vi "Facade.vi"(0 "Data In":T4, 2 "Display State In":T2, 3 "Container State":T3) -> (6 "Data Out":T4, 7 "Display State Out":T2, 8 "Action":T1)   [LabVIEW 2009, in "HistoryPath.xctl"]
uses:
  HistoryPath.xctl
  Data.ctl
  <vilib>/_xctls/Container State.ctl
  State.ctl
  <vilib>/_xctls/Action.ctl
  <vilib>/_xctls/XControlSupport.lvlib
panel:
  in  "Browse":bool
  in  "Combo Box":string(combo)
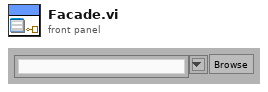
[diagram p1: front panel]
types:
  T1 = typedef "XControlSupport.lvlib/Action.ctl" = cluster{"Data Changed?":bool, "State Changed?":bool, "Action Name":string}
  T2 = typedef "HistoryPath.xctl/State.ctl" = cluster{"History":path[], "History Length":i32}
  T3 = typedef "XControlSupport.lvlib/Container State.ctl" = cluster{"Indicator?":bool, "Run Mode?":bool, " Refnum":refnum<vi>}
  T4 = typedef "HistoryPath.xctl/Data.ctl" = path
  T5 = enum8{"Enabled", "Disabled", "Disabled and Grayed Out"}
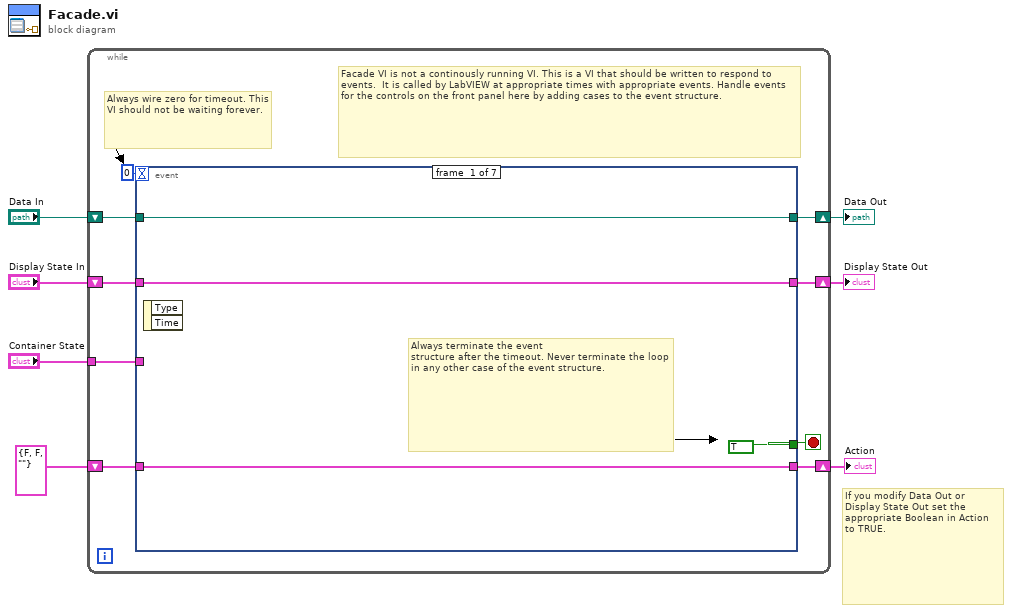
[diagram p0: block diagram]
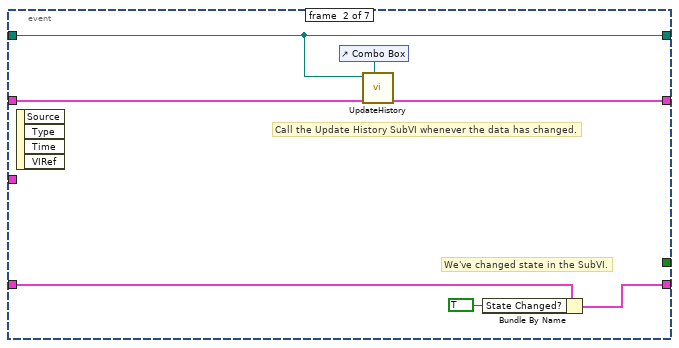
[diagram p2: hidden frame]
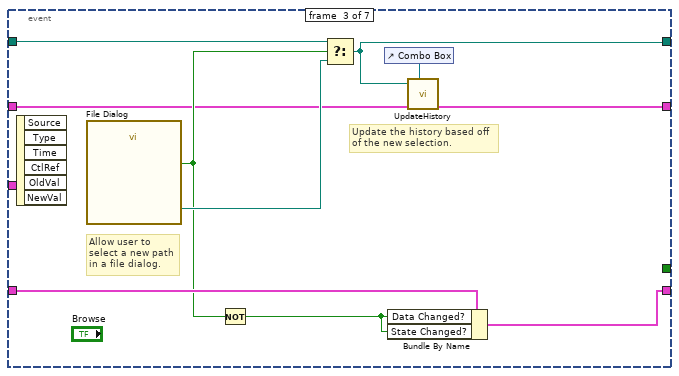
[diagram p3: hidden frame]
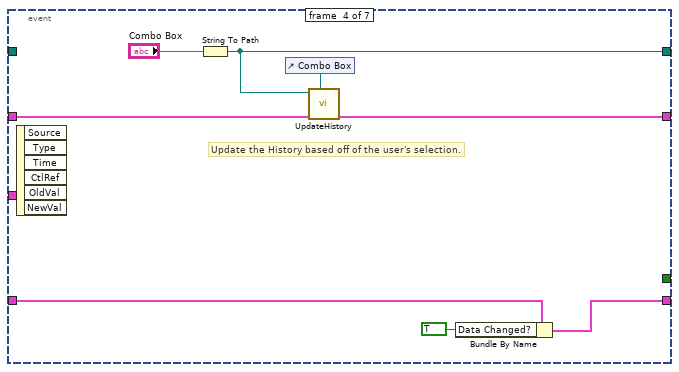
[diagram p4: hidden frame]
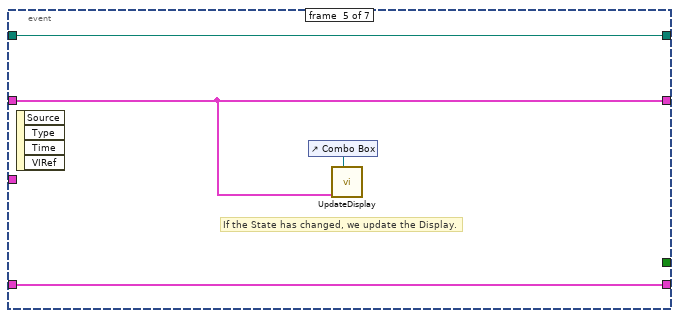
[diagram p5: hidden frame]
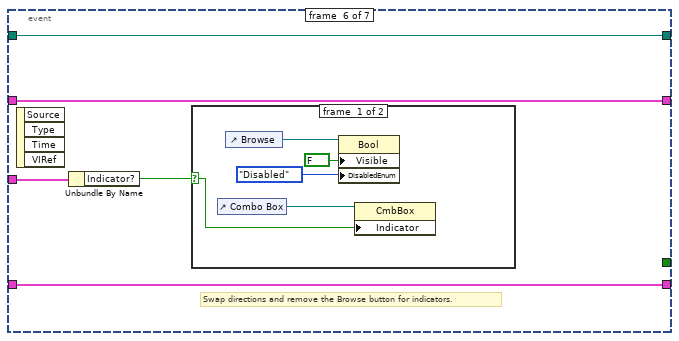
[diagram p6: hidden frame]
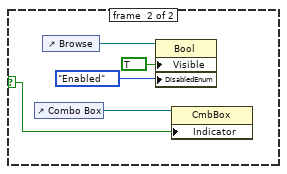
[diagram p7: hidden frame]
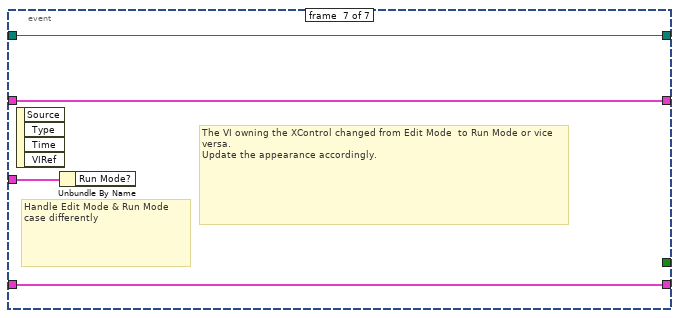
[diagram p8: hidden frame]
diagram:
  # "If you modify Data Out or\nDisplay State Out set the\nappropriate Boolean in Action\nto TRUE."
  n1 = while {
    shift-right: [w15] -> w4
    shift-left: "Display State In" -> [w16]
    tunnel: "Container State" -> [w12]
    shift-right: [w10] -> w7
    shift-left: "Data In" -> [w11]
    shift-right: [w8] -> w2
    shift-left: T1 {"Data Changed?"=FALSE, "State Changed?"=FALSE, "Action Name"=""} ("Action") -> [w9]
    stop <- w14 stop-if-true
    # "Facade VI is not a continously running VI. This is a VI that should be written to respond to events.  It is called by LabVIEW at appropriate times with appropriate events. Handle events for the controls on the front panel here by adding cases to the event structure."
    # "Always wire zero for timeout. This\nVI should not be waiting forever."
    n2 = event shown="[2] \"Browse\": Value Change" {
      selector: _ -> [_ _ _ _ _ _ _]
      dyn-events: _ -> [_ _ _ _ _ _ _]
      timeout: 0 -> [_ _ _ _ _ _ _]
      tunnel: w16 -> [w18 w27 w32 w40 w47 w53 w67]
      tunnel: [w18 w22 w30 w39 w47 w53 w67] -> w15
      tunnel: [TRUE _ _ _ _ _ _] -> w14
      tunnel: w12 -> [_ _ _ _ _ w54 w68]
      tunnel: w11 -> [w17 w23 w35 _ w49 w52 w66]
      tunnel: [w17 w23 w31 w38 w49 w52 w66] -> w10
      tunnel: [w19 w26 w36 w43 w48 w51 w65] -> w8
      tunnel: w9 -> [w19 w25 w37 w44 w48 w51 w65]
      event #0 {
        # "Always terminate the event\nstructure after the timeout. Never terminate the loop in any other case of the event structure."
        n3 = event-data() -> ()  [unwired: 1 in, 2 out]
      }
      event #1 {
        # "We've changed state in the SubVI."
        # "Call the Update History SubVI whenever the data has changed."
        n4 = event-data() -> ()  [unwired: 1 in, 4 out]
        n5 = control-ref of="Combo Box"() -> (w21:refnum<vi>)
        n6 = call "UpdateHistory.vi"("CmbBox Refnum"=w21, "Display State In 2"=w27, "Data In"=w23) -> ("Display State In"=w22:T2)  [unwired: 8 in]
        n7 = Bundle By Name(cluster=w25, "State Changed?"=TRUE) -> (w26:T1)
      }
      event #2 {
        # "Update the history based off of the new selection."
        # "Allow user to select a new path in a file dialog."
        n8 = event-data() -> ()  [unwired: 1 in, 6 out]
        n9 = call "File Dialog"() -> ("selected path"=w34:path, "cancelled"=w33:bool)  [unwired: 12 in, 2 out]
        n10 = Not(x=w33) -> (.not. x?=w28:bool)
        n11 = Select(t=w35, s=w33, f=w34) -> (s? t:f=w31:T4)
        n12 = control-ref of="Combo Box"() -> (w29:refnum<vi>)
        n13 = Bundle By Name(cluster=w37, "Data Changed?"=w28, "State Changed?"=w28) -> (w36:T1)
        n14 = call "UpdateHistory.vi"("CmbBox Refnum"=w29, "Display State In 2"=w32, "Data In"=w31) -> ("Display State In"=w30:T2)  [unwired: 8 in]
      }
      event #3 {
        # "Update the History based off of the user's selection."
        n15 = event-data() -> ()  [unwired: 1 in, 6 out]
        n16 = String To Path(string="Combo Box") -> (path=w38:path)
        n17 = control-ref of="Combo Box"() -> (w41:refnum<vi>)
        n18 = call "UpdateHistory.vi"("CmbBox Refnum"=w41, "Display State In 2"=w40, "Data In"=w38) -> ("Display State In"=w39:T2)  [unwired: 8 in]
        n19 = Bundle By Name(cluster=w44, "Data Changed?"=TRUE) -> (w43:T1)
      }
      event #4 {
        # "If the State has changed, we update the Display."
        n20 = event-data() -> ()  [unwired: 1 in, 4 out]
        n21 = control-ref of="Combo Box"() -> (w46:refnum<vi>)
        n22 = call "UpdateDisplay.vi"("CmbBox Refnum"=w46, "Display State In"=w47) -> ()  [unwired: 10 in]
      }
      event #5 {
        # "Swap directions and remove the Browse button for indicators."
        n23 = event-data() -> ()  [unwired: 1 in, 4 out]
        n24 = Unbundle By Name(w54) -> ("Indicator?"=w50:bool)
        n25 = case shown="False" w50 {
          selector: w50 -> [w58 w63]
          frame #0 {
            n26 = control-ref of="Combo Box"() -> (w59:refnum<vi>)
            n27 = control-ref of="Browse"() -> (w57:refnum<vi>)
            n28 = property class="Bool"(reference=w57, "Visible"=FALSE, "DisabledEnum"=T5."Disabled" ("Disabled")) -> ()  [unwired: 1 in, 2 out]
            n29 = property class="CmbBox"(reference=w59, "Indicator"=w58) -> ()  [unwired: 1 in, 2 out]
          }
          frame #1 {
            n30 = control-ref of="Combo Box"() -> (w64:refnum<vi>)
            n31 = control-ref of="Browse"() -> (w62:refnum<vi>)
            n32 = property class="Bool"(reference=w62, "Visible"=TRUE, "DisabledEnum"=T5."Enabled" ("Disabled")) -> ()  [unwired: 1 in, 2 out]
            n33 = property class="CmbBox"(reference=w64, "Indicator"=w63) -> ()  [unwired: 1 in, 2 out]
          }
        }
      }
      event #6 {
        # "The VI owning the XControl changed from Edit Mode  to Run Mode or vice versa.\nUpdate the appearance accordingly."
        # "Handle Edit Mode & Run Mode\ncase differently"
        n34 = event-data() -> ()  [unwired: 1 in, 4 out]
        n35 = Unbundle By Name(w68) -> ()  [unwired: 1 out]
      }
    }
  }
  "Display State Out" <- w4
  "Data Out" <- w7
  "Action" <- w2
